vi "Read Description.vi"(11 "Espresso in":refnum<class "Espresso.lvclass">) -> (2 "Description":string)   [LabVIEW 2013, in "Espresso.lvclass"]
uses:
  Espresso.lvclass
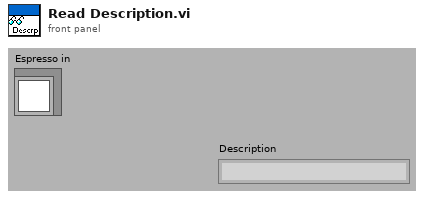
[diagram p1: front panel]
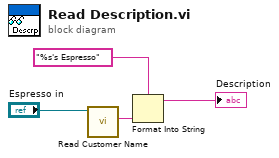
[diagram p0: block diagram]
diagram:
  n1 = call-dynamic "Read Customer Name.vi"("Beverage in"="Espresso in") -> ("Customer Name"=w4:string)  [unwired: 10 in]
  n2 = Format Into String(format string="%s's Espresso" ("Description"), w4) -> (resulting string=→"Description":string)  [unwired: 2 in, 1 out]
